vi "myRIO_BRig_FPGA_v3,71.vi"() -> ()   [LabVIEW 2014]
uses:
  <vilib>/rvi/Emulation/niFpgaGetClockAttributes.vi
  <vilib>/rvi/Emulation/niFpgaSctlEmulationGetInTimedLoop.vi
  <vilib>/rvi/Emulation/niFpgaEmulationReportErrorSimple.vi
  <vilib>/rvi/eio/common/nirviEmuTemplateMethod_errors.vi
  <vilib>/rvi/Emulation/niFpgaCriticalErrorInLSC.vi
  <vilib>/eio/EIONode/EIONode.xnode
panel:
  in  "AnaOut_1":u16
  in  "CueLed_Event":bool
  in  "CueLed_nValley":u32=100
  in  "CueLed_nPeak":u32=100
  in  "LC_Event_l2":bool
  in  "LC_Laser_l2":bool
  in  "LC_nShutter_l2":u32=100
  in  "LC_nValley_l2":u32=100
  in  "LC_nPeak_l2":u32=100
  in  "LR_wrong_nDelay_l2":u32
  in  "LR_reward_nDelay_l2":u32
  in  "LR_wrong_nTotal_l2":u32=100
  in  "LR_reward_nTotal_l2":u32=100
  in  "LR_wrong_laser_l2":bool
  in  "LR_wrong_Event_l2":bool
  in  "LR_reward_Laser_l2":bool
  in  "LR_reward_Event_l2":bool
  out "AnaIn_1":u16
  out "AnaIn_0":u16
  out "timeTrial_count":u32
  in  "timeTrial_trig":bool
  in  "k1__counter_per_ms":u16=100 min=100 max=40000 step=1
  in  "LC_nShutter_l1":u32=100
  in  "AnaOut_0":u16
  in  "LC_nValley_l1":u32=100
  in  "LC_nPeak_l1":u32=100
  in  "LC_Event_l1":bool
  in  "LR_wrong_nTotal_l1":u32=100
  in  "LR_wrong_nDelay_l1":u32
  in  "LR_reward_nTotal_l1":u32=100
  in  "LR_reward_nDelay_l1":u32
  in  "LR_reward_Event_l1":bool
  in  "LR_wrong_Event_l1":bool
  out "SelectWrong":bool
  out "SelectReward":bool
  in  "LR_wrong_Laser_l1":bool
  in  "LR_reward_Laser_l1":bool
  in  "Left(F)_or_Right(T)":bool
  in  "ignoreWrong":bool
  in  "SelectionState":bool
  in  "LC_Laser_l1":bool
  in  "FPGA_Stop":bool
  in  "audioTrigger_L":bool
  in  "audioTrigger_R":bool
  in  "audioFreq_L_kHz":u8=14 min=1 max=14 step=1
  in  "audioAmp_L":u16=1 min=1 max=32767 step=1
  in  "audioFreq_R_kHz":u8=14 min=1 max=14 step=1
  in  "audioAmp_R":u16=1 min=1 max=32767 step=1
  in  "A3_SL":bool
  in  "A1_SR":bool
  in  "Counts_Reset":bool
  out "A4_LickR":u32
  out "A2_LickL":u32
  in  "A6_Act":bool
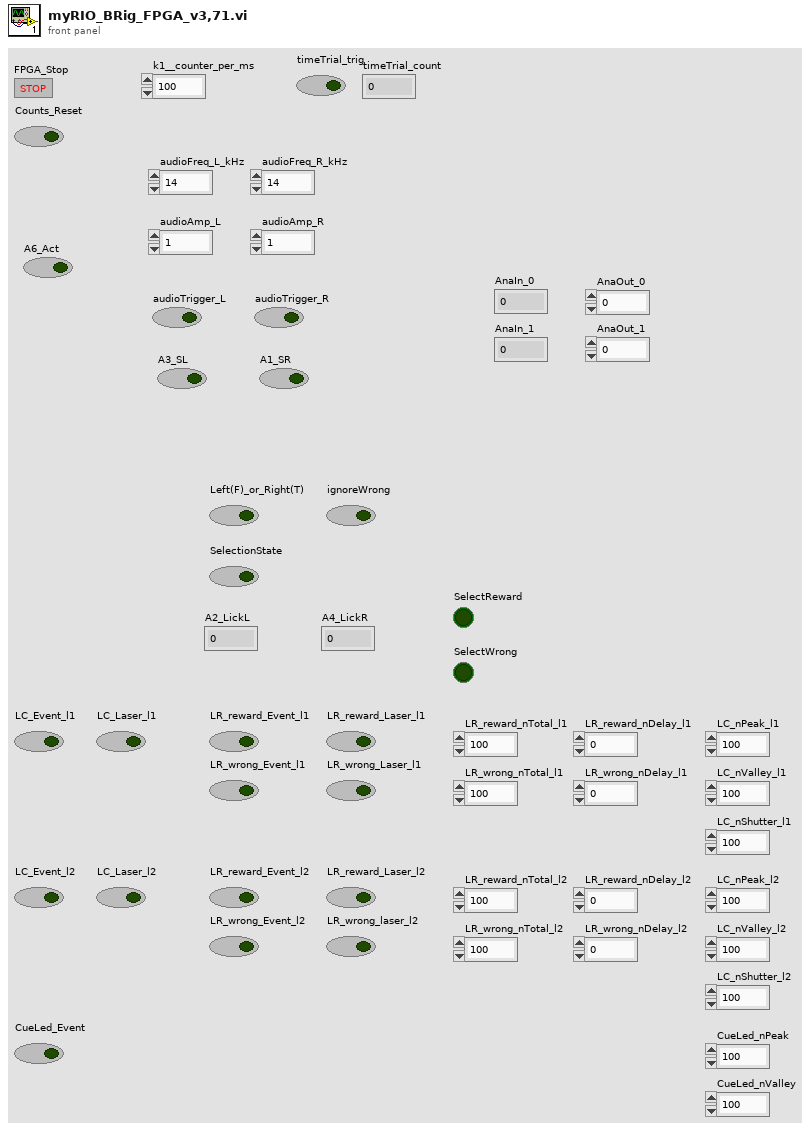
[diagram p1: front panel]
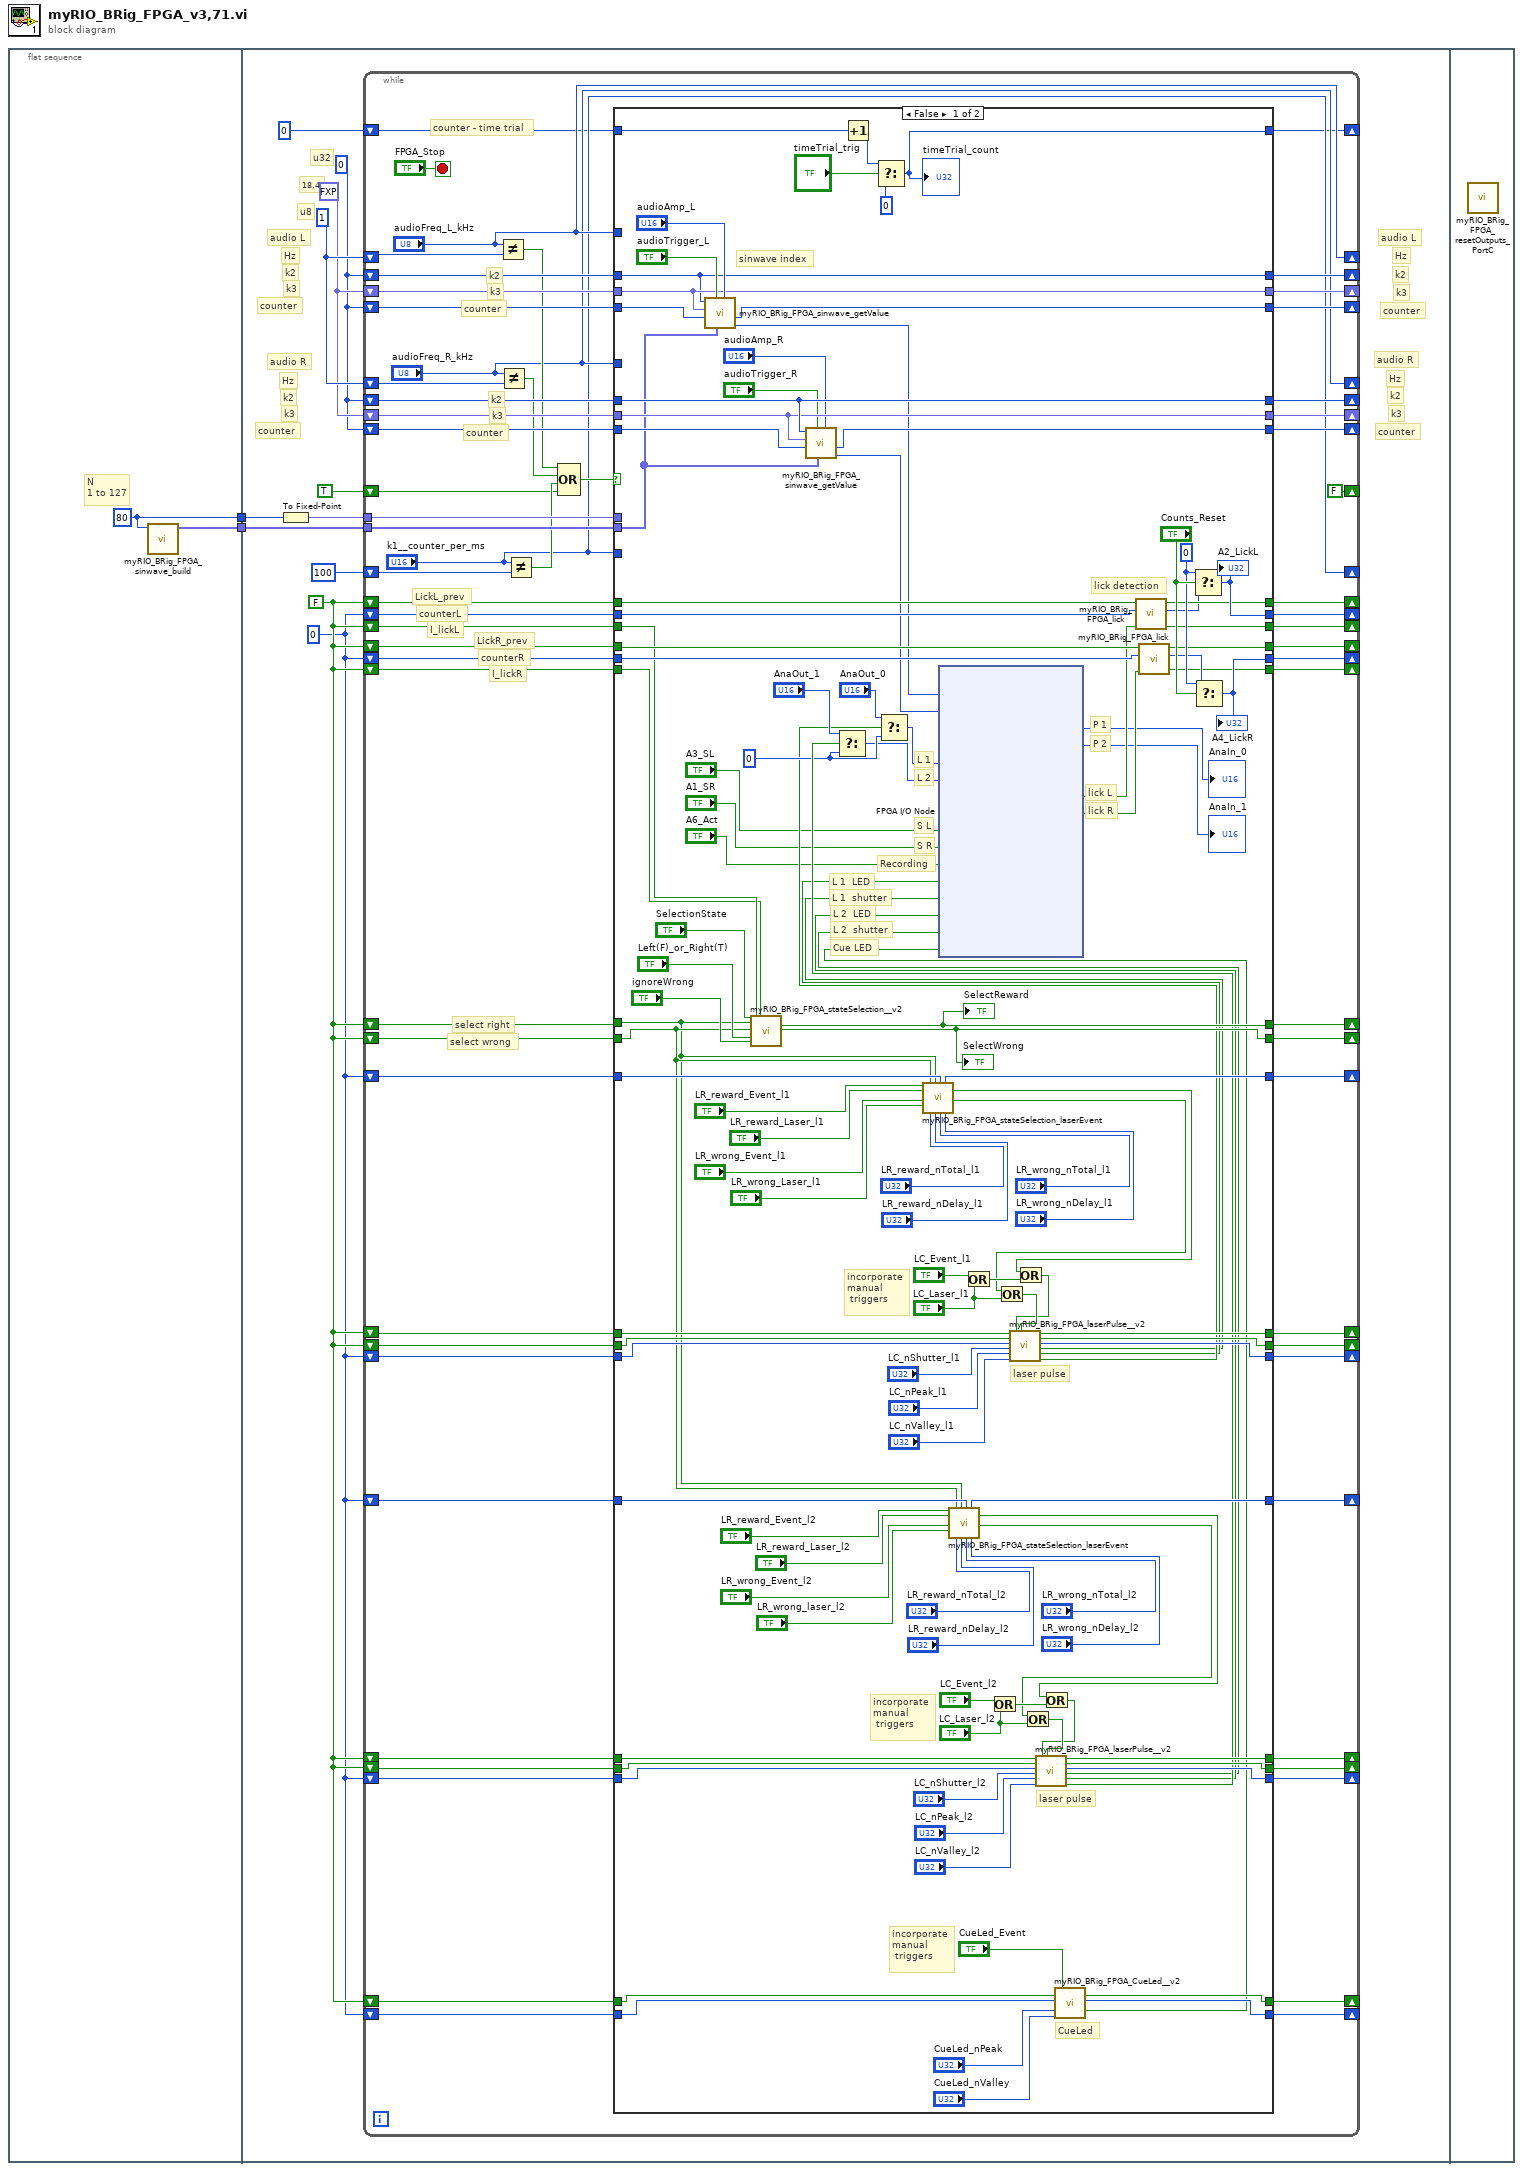
[diagram p0: block diagram]
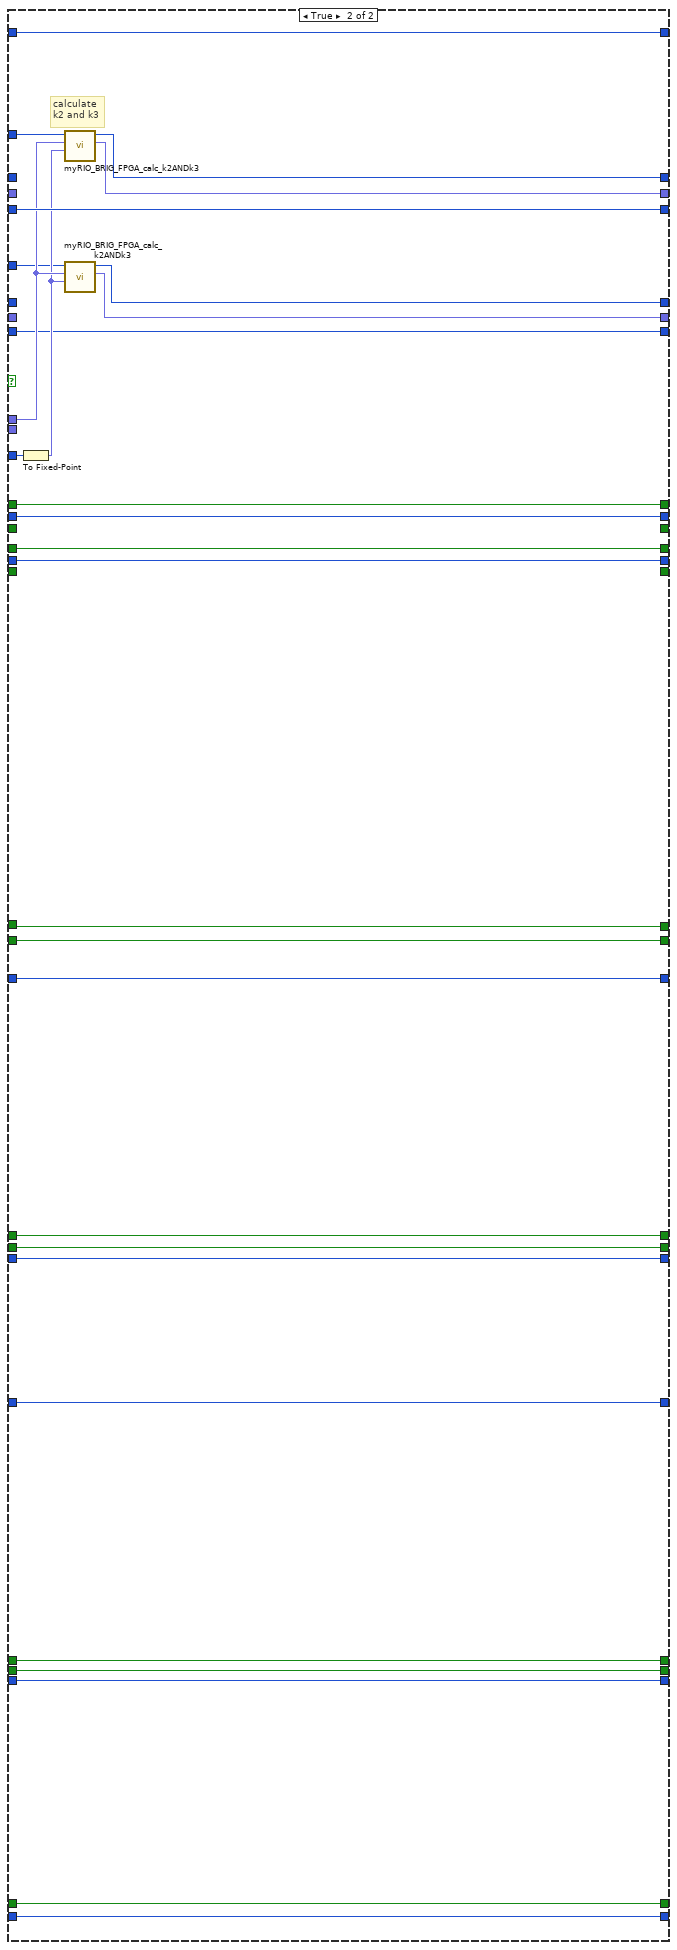
[diagram p2: hidden frame]
diagram:
  n1 = flat-sequence {
    tunnel: [w4] -> w2
    tunnel: [w3] -> w1
    tunnel: w2 -> [w15]
    tunnel: w1 -> [w14]
    frame #0 {
      w3 = 80 ("dimension size")
      # "N\n1 to 127"
      n2 = call "myRIO_BRig_FPGA_sinwave_build.vi"("input_Npts"=w3) -> ("output_array_sin"=w4:fxp<+/-,16,2>[])  [unwired: 10 in]
    }
    frame #1 {
      w5 = u32 0
      w6 = FALSE
      w10 = u32 0
      w11 = fxp<+,18,4> 0.0
      w12 = u8 1
      # "counter"
      # "k3"
      # "k2"
      # "counter"
      # "k3"
      # "k2"
      # "counter"
      # "counter"
      # "u32"
      # "k3"
      # "k2"
      # "k3"
      # "18,4"
      # "u8"
      # "Hz"
      # "Hz"
      # "audio R"
      # "audio L"
      # "Hz"
      # "k2"
      # "Hz"
      # "audio R"
      # "audio L"
      n3 = To Fixed-Point(number=w14) -> (fixed-point=w13:fxp<+,7,7>)  [unwired: 1 in]
      n4 = while {
        shift-right: ["audioFreq_L_kHz"] -> _
        shift-left: w12 -> [w80]
        shift-right: [w74] -> _
        shift-left: w10 -> [w78]
        shift-right: ["audioFreq_R_kHz"] -> _
        shift-left: w12 -> [w70]
        tunnel: w15 -> [w77]
        tunnel: w13 -> [w76]
        shift-right: [w73] -> _
        shift-left: w11 -> [w75]
        shift-right: [w71] -> _
        shift-left: w10 -> [w72]
        shift-right: [w68] -> _
        shift-left: w10 -> [w69]
        shift-right: [w66] -> _
        shift-left: w11 -> [w67]
        shift-right: [w64] -> _
        shift-left: w10 -> [w65]
        shift-right: ["k1__counter_per_ms"] -> _
        shift-left: u16 100 ("y") -> [w63]
        shift-right: [FALSE] -> _
        shift-left: TRUE -> [w58]
        shift-right: [w51] -> _
        shift-left: w6 -> [w53]
        shift-right: [w50] -> _
        shift-left: w6 -> [w52]
        shift-right: [w48] -> _
        shift-left: w5 -> [w49]
        shift-right: [w46] -> _
        shift-left: w5 -> [w47]
        shift-right: [w43] -> _
        shift-left: w6 -> [w45]
        shift-right: [w42] -> _
        shift-left: w6 -> [w44]
        shift-right: [w40] -> _
        shift-left: w6 -> [w41]
        shift-right: [w38] -> _
        shift-left: w6 -> [w39]
        shift-right: [w36] -> _
        shift-left: u32 0 -> [w37]
        shift-right: [w34] -> _
        shift-left: w5 -> [w35]
        shift-right: [w33] -> _
        shift-left: w6 -> [w30]
        shift-right: [w32] -> _
        shift-left: w6 -> [w29]
        shift-right: [w31] -> _
        shift-left: w5 -> [w28]
        shift-right: [w26] -> _
        shift-left: w5 -> [w27]
        shift-right: [w25] -> _
        shift-left: w6 -> [w22]
        shift-right: [w24] -> _
        shift-left: w6 -> [w21]
        shift-right: [w23] -> _
        shift-left: w5 -> [w20]
        shift-right: [w19] -> _
        shift-left: w6 -> [w17]
        shift-right: [w18] -> _
        shift-left: w5 -> [w16]
        stop <- "FPGA_Stop" stop-if-true
        # "counter"
        # "k3"
        # "k2"
        # "counter"
        # "k3"
        # "k2"
        # "counter - time trial"
        # "I_lickR"
        # "counterR"
        # "LickR_prev"
        # "I_lickL"
        # "counterL"
        # "LickL_prev"
        # "select wrong"
        # "select right"
        n5 = Not Equal?(x="audioFreq_L_kHz", y=w80) -> (x != y?=w62:bool)
        n6 = Not Equal?(x="audioFreq_R_kHz", y=w70) -> (x != y?=w61:bool)
        n7 = Not Equal?(x="k1__counter_per_ms", y=w63) -> (x != y?=w59:bool)
        n8 = Compound Arithmetic op=OR(w62, w61, w59, w58) -> (w60:bool)
        n9 = case shown="False" w60 {
          tunnel: w78 -> [w186 _]
          tunnel: "audioFreq_L_kHz" -> [_ w228]
          tunnel: w77 -> [w179 _]
          tunnel: w76 -> [_ w224]
          tunnel: "k1__counter_per_ms" -> [_ w229]
          tunnel: w75 -> [w187 _]
          tunnel: [w186 w227] -> w74
          tunnel: [w187 w226] -> w73
          tunnel: w72 -> [w191 w225]
          tunnel: [w188 w225] -> w71
          tunnel: w69 -> [w183 _]
          tunnel: [w183 w220] -> w68
          tunnel: w67 -> [w182 _]
          tunnel: [w182 w221] -> w66
          tunnel: w65 -> [w185 w219]
          tunnel: "audioFreq_R_kHz" -> [_ w222]
          tunnel: [w184 w219] -> w64
          tunnel: w53 -> [w174 w218]
          tunnel: w52 -> [w173 w217]
          tunnel: [w178 w218] -> w51
          tunnel: [w171 w217] -> w50
          tunnel: w49 -> [w175 w216]
          tunnel: [w201 w216] -> w48
          tunnel: w47 -> [w172 w215]
          tunnel: [w198 w215] -> w46
          tunnel: w45 -> [w111 w214]
          tunnel: w44 -> [w112 w213]
          tunnel: [w147 w214] -> w43
          tunnel: [w194 w213] -> w42
          tunnel: [w164 w210] -> w33
          tunnel: [w165 w209] -> w32
          tunnel: [w166 w208] -> w31
          tunnel: w41 -> [w168 _]
          tunnel: [w177 _] -> w40
          tunnel: w39 -> [w167 _]
          tunnel: [w169 _] -> w38
          tunnel: w37 -> [w156 w212]
          tunnel: [w153 w212] -> w36
          tunnel: w35 -> [w146 w211]
          tunnel: [w145 w211] -> w34
          tunnel: w30 -> [w136 w210]
          tunnel: w29 -> [w135 w209]
          tunnel: w28 -> [w134 w208]
          tunnel: w27 -> [w116 w207]
          tunnel: [w115 w207] -> w26
          tunnel: [w109 w206] -> w25
          tunnel: [w108 w205] -> w24
          tunnel: [w107 w204] -> w23
          tunnel: w22 -> [w106 w206]
          tunnel: w21 -> [w105 w205]
          tunnel: w20 -> [w104 w204]
          tunnel: [w101 w203] -> w19
          tunnel: [w100 w202] -> w18
          tunnel: w17 -> [w99 w203]
          tunnel: w16 -> [w98 w202]
          frame False {
            w94 = u16 0 ("f")
            w199 = u32 0 ("t")
            # "Cue LED"
            # "L 2  shutter"
            # "L 2  LED"
            # "L 1  shutter"
            # "L 1  LED"
            # "Recording"
            # "P 2"
            # "P 1"
            # "L 2"
            # "L 1"
            # "S L"
            # "S R"
            # "lick R"
            # "lick L"
            # "CueLed"
            # "incorporate\nmanual\n triggers"
            # "laser pulse"
            # "incorporate\nmanual\n triggers"
            # "sinwave index"
            # "lick detection"
            # "laser pulse"
            # "incorporate\nmanual\n triggers"
            n10 = call "myRIO_BRig_FPGA_sinwave_getValue.vi"("audioAmp"="audioAmp_L", "sinwave"=w179, "audioTrigger"="audioTrigger_L", "counter"=w191, "k3"=w187, "k2"=w186) -> ("output_audioValue"=w151:i16, "output_counter"=w188:u32)  [unwired: 4 in]
            n11 = call "myRIO_BRig_FPGA_stateSelection__v2.vi"("I_selectionState"="SelectionState", "I_selectRight"=w111, "I_selectWrong"=w112, "I_Left(F)_or_Right(T)"="Left(F)_or_Right(T)", "I_ignoreWrong"="ignoreWrong", "I_lickL"=w168, "I_lickR"=w167) -> ("output__I_selectRight"=w147:bool, "output__I_selectWrong"=w194:bool)  [unwired: 19 in]
            "SelectWrong" <- w194
            "SelectReward" <- w147
            n12 = call "myRIO_BRig_FPGA_sinwave_getValue.vi"("audioAmp"="audioAmp_R", "sinwave"=w179, "audioTrigger"="audioTrigger_R", "counter"=w185, "k3"=w182, "k2"=w183) -> ("output_audioValue"=w150:i16, "output_counter"=w184:u32)  [unwired: 4 in]
            n13 = Increment(x=w156) -> (x+1=w155:u32)
            n14 = Select(t=w155, s="timeTrial_trig", f=u32 0) -> (s? t:f=w153:u32)
            "timeTrial_count" <- w153
            n15 = call "myRIO_BRig_FPGA_stateSelection_laserEvent.vi"("I_LR_reward"="LR_reward_Event_l1", "I_LR_reward_laser"="LR_reward_Laser_l1", "I_LR_wrong"="LR_wrong_Event_l1", "I_LR_wrong_laser"="LR_wrong_Laser_l1", "I_selectWrong"=w112, "laser_reward_nTotal"="LR_reward_nTotal_l1", "I_selectReward"=w111, "laser_reward_nDelay"="LR_reward_nDelay_l1", "counter"=w146, "laser_wrong_nTotal"="LR_wrong_nTotal_l1", "laser_wrong_nDelay"="LR_wrong_nDelay_l1") -> ("output_counter"=w145:u32, "output_I_laserEvent"=w133:bool, "output_I_laserOn"=w132:bool)  [unwired: 6 in]
            n16 = call "myRIO_BRig_FPGA_stateSelection_laserEvent.vi"("I_LR_reward"="LR_reward_Event_l2", "I_LR_reward_laser"="LR_reward_Laser_l2", "I_LR_wrong"="LR_wrong_Event_l2", "I_LR_wrong_laser"="LR_wrong_laser_l2", "I_selectWrong"=w112, "laser_reward_nTotal"="LR_reward_nTotal_l2", "I_selectReward"=w111, "laser_reward_nDelay"="LR_reward_nDelay_l2", "counter"=w116, "laser_wrong_nTotal"="LR_wrong_nTotal_l2", "laser_wrong_nDelay"="LR_wrong_nDelay_l2") -> ("output_counter"=w115:u32, "output_I_laserEvent"=w110:bool, "output_I_laserOn"=w117:bool)  [unwired: 6 in]
            n17 = Or(x="LC_Event_l1", y="LC_Laser_l1") -> (x .or. y?=w160:bool)
            n18 = Or(x="LC_Event_l2", y="LC_Laser_l2") -> (x .or. y?=w127:bool)
            n19 = Or(x=w132, y="LC_Laser_l1") -> (x .or. y?=w158:bool)
            n20 = Or(x=w133, y=w160) -> (x .or. y?=w157:bool)
            n21 = call "myRIO_BRig_FPGA_laserPulse__v2.vi"("I_shutter"=w136, "I_peak"=w135, "count"=w134, "laser_Nshutter"="LC_nShutter_l1", "laser_Npeak"="LC_nPeak_l1", "laser_Nvalley"="LC_nValley_l1", "I_laserEvent"=w157, "I_laser"=w158) -> ("output_I_shutter"=w164:bool, "output_I_peak"=w165:bool, "output_count"=w166:u32, "output_shutter"=w84:bool, "output_led"=w85:bool, "output_laser"=w92:bool)  [unwired: 6 in]
            n22 = Select(t="AnaOut_0", s=w92, f=w94) -> (s? t:f=w96:u16)
            n23 = Or(x=w117, y="LC_Laser_l2") -> (x .or. y?=w125:bool)
            n24 = Or(x=w110, y=w127) -> (x .or. y?=w124:bool)
            n25 = call "myRIO_BRig_FPGA_laserPulse__v2.vi"("I_shutter"=w106, "I_peak"=w105, "count"=w104, "laser_Nshutter"="LC_nShutter_l2", "laser_Npeak"="LC_nPeak_l2", "laser_Nvalley"="LC_nValley_l2", "I_laserEvent"=w124, "I_laser"=w125) -> ("output_I_shutter"=w109:bool, "output_I_peak"=w108:bool, "output_count"=w107:u32, "output_shutter"=w81:bool, "output_led"=w82:bool, "output_laser"=w95:bool)  [unwired: 6 in]
            n26 = Select(t="AnaOut_1", s=w95, f=w94) -> (s? t:f=w91:u16)
            n27 = call "myRIO_BRig_FPGA_CueLed__v2.vi"("I_peak"=w99, "count"=w98, "laser_Npeak"="CueLed_nPeak", "laser_Nvalley"="CueLed_nValley", "I_CueLed_Event"="CueLed_Event") -> ("output_I_peak"=w101:bool, "output_count"=w100:u32, "output_led"=w83:bool)  [unwired: 12 in]
            n28 = xnode "FPGA I/O Node"("AudioOut/Left"=w151, "AudioOut/Right"=w150, "ConnectorB/AO0"=w96, "ConnectorB/AO1"=w91, "ConnectorA/DIO3"="A3_SL", "ConnectorA/DIO5"="A1_SR", "ConnectorA/DIO0"="A6_Act", "ConnectorA/DIO14"=w85, "ConnectorA/DIO6"=w84, "ConnectorA/DIO12"=w82, "ConnectorA/DIO7"=w81, "ConnectorA/DIO9"=w83) -> ("ConnectorB/AI1"=→"AnaIn_0":u16, "ConnectorB/AI2"=→"AnaIn_1":u16, "ConnectorA/DIO4"=w149:bool, "ConnectorA/DIO2"=w148:bool)  [unwired: 16 in, 16 out]
            n29 = call "myRIO_BRig_FPGA_lick.vi"("I_stateDetector_new"=w149, "counter"=w175, "I_stateDetector_prev"=w174) -> ("output_I_lick"=w177:bool, "output_counter"=w176:u32, "output_I_stateDetector_prev"=w178:bool)  [unwired: 6 in]
            n30 = call "myRIO_BRig_FPGA_lick.vi"("I_stateDetector_new"=w148, "counter"=w172, "I_stateDetector_prev"=w173) -> ("output_I_lick"=w169:bool, "output_counter"=w170:u32, "output_I_stateDetector_prev"=w171:bool)  [unwired: 6 in]
            n31 = Select(t=w199, s="Counts_Reset", f=w176) -> (s? t:f=w201:u32)
            "A2_LickL" <- w201
            n32 = Select(t=w199, s="Counts_Reset", f=w170) -> (s? t:f=w198:u32)
            "A4_LickR" <- w198
          }
          frame True {
            # "calculate\nk2 and k3"
            n33 = To Fixed-Point(number=w229) -> (fixed-point=w223:fxp<+,16,16>)  [unwired: 1 in]
            n34 = call "myRIO_BRIG_FPGA_calc_k2ANDk3.vi"("input_k1[count/ms]"=w223, "input_Npts"=w224, "input_freq[kHz]"=w228) -> ("output_k3"=w226:fxp<+,18,4>, "output_k2"=w227:u32)  [unwired: 7 in]
            n35 = call "myRIO_BRIG_FPGA_calc_k2ANDk3.vi"("input_k1[count/ms]"=w223, "input_Npts"=w224, "input_freq[kHz]"=w222) -> ("output_k3"=w221:fxp<+,18,4>, "output_k2"=w220:u32)  [unwired: 7 in]
          }
        }
      }
    }
    frame #2 {
      n36 = call "myRIO_BRig_FPGA_resetOutputs_PortC.vi"() -> ()  [unwired: 12 in]
    }
  }
